vi "Tear Down.vi"(8 "error in (no error)":errorcluster, 11 "Car Wash Station Sequencer in":refnum<class "Car Wash Station Sequencer.lvclass">) -> (0 "error out":errorcluster, 3 "Car Wash Station Sequencer out":refnum<class "Car Wash Station Sequencer.lvclass">)   [LabVIEW 2016, in "CLD Exam - Car Wash.lvlib" / "Car Wash Station Sequencer.lvclass"]
uses:
  Car Wash Station Sequencer.lvclass
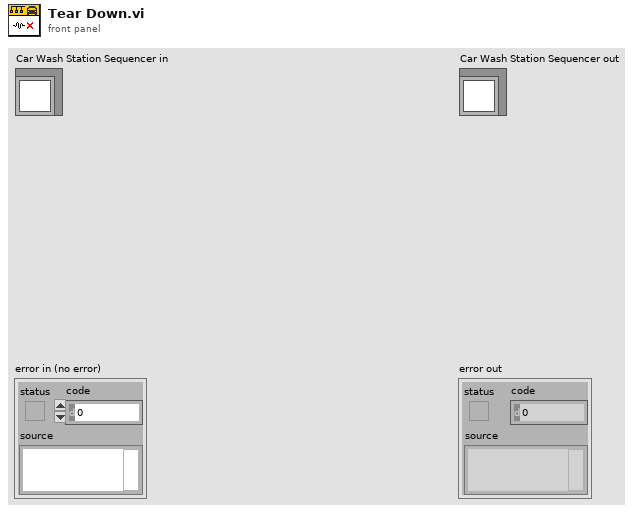
[diagram p1: front panel]
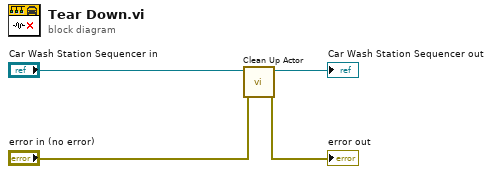
[diagram p0: block diagram]
diagram:
  n1 = call-dynamic "Clean Up Actor.vi"("error in (no error)"="error in (no error)", "Car Wash Station Sequencer in"="Car Wash Station Sequencer in") -> ("error out"=→"error out":errorcluster, "Car Wash Station Sequencer out"=→"Car Wash Station Sequencer out":refnum<class "Car Wash Station Sequencer.lvclass">)  [unwired: 8 in]
